vi "Manual Assembly DB.vi"() -> ()   [LabVIEW 2021]
uses:
  Classes/Routine/Routine Enum.ctl
  Classes/Assembly/Database Entry/Database Entry.lvclass
  Classes/Assembly/Assembly Run.lvclass
  Classes/Workspace/Fixture Enum.ctl
  <vilib>/Utility/file.llb/Read Delimited Spreadsheet (string).vi
  SubVIs/PUT_region.vi
  SubVIs/component_tray_region.vi
  SubVIs/assembly_tray_region.vi
  Classes/Workspace/Fixture.lvclass
  Classes/Controller/Controller.lvclass
  <vilib>/JDP Science/JDP Science Common Utilities/JDP Utility.lvlib
  Classes/Routine/Routine.lvclass
panel:
  out "Assembly Type":string[](array[string])
  out "Assembly tray region":dbl
  out "Component tray region":dbl
  out "PUT Region":dbl
  in  "Clear All":bool
  in  "Assemble":bool
  in  "Pick and Place":bool
  in  "Dispense glue":bool
  in  "Go":bool
  in  "Routine":T1=enum."Dispense Epoxy"
  in  "Update":bool
  in  "Stage":i32(listbox)=-1
  in  "Stop":bool
  in  "Remove":bool
  in  "Add":bool
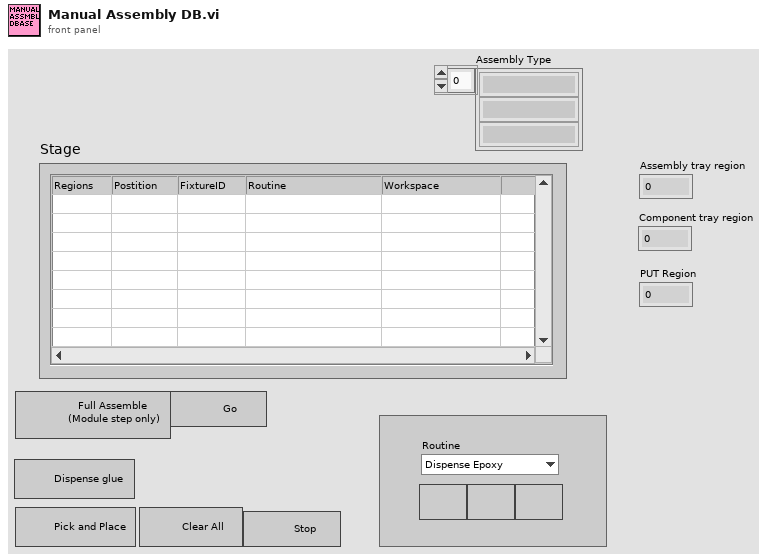
[diagram p1: front panel]
types:
  T1 = typedef "Routine.lvclass/Routine Enum.ctl" = enum16{"Primary Pick Up", "Secondary Pick Up", "Put Down All", "Secure Syringe", "Release Syringe", "Dispense Epoxy", "Pick Up All", "Put Down Secondary", "Full Assembly"}
  T2 = typedef "Fixture.lvclass/Fixture Enum.ctl" = enum16{"Assembly Tray", "Syringe Space", "Component", "Pick Up Tool", "Current Position"}
  T3 = typedef "File Paths.ctl" = cluster{"Glue Pattern Folder":path, "Carrier Tray Folder":path, "Pick Up Tool Fixture Folder":path, "Components Folder":path, "Bellows Tool Offset.txt":path, "Pick Up Tool Offset.txt":path, "Dispense Tip Offset.txt":path, "Log Files":path, "Gantry Assembly Map.txt":path, "Syringe and offset map.txt":path, "Controllers Folder":path, "Local dbase config":path}
  T4 = cluster{"Fixture ID":dbl, "Position":dbl, "Thickness":dbl}[]
  T5 = typedef "Controller.lvclass/Controllers.ctl" = cluster{"I-O.lvclass":refnum<class "I-O.lvclass">, "Gantry":refnum<k24>, "Dispenser":refnum<visa-resource-name>}
  T6 = cluster{"Fixture ID":dbl, "Position":dbl, "Thickness":dbl}
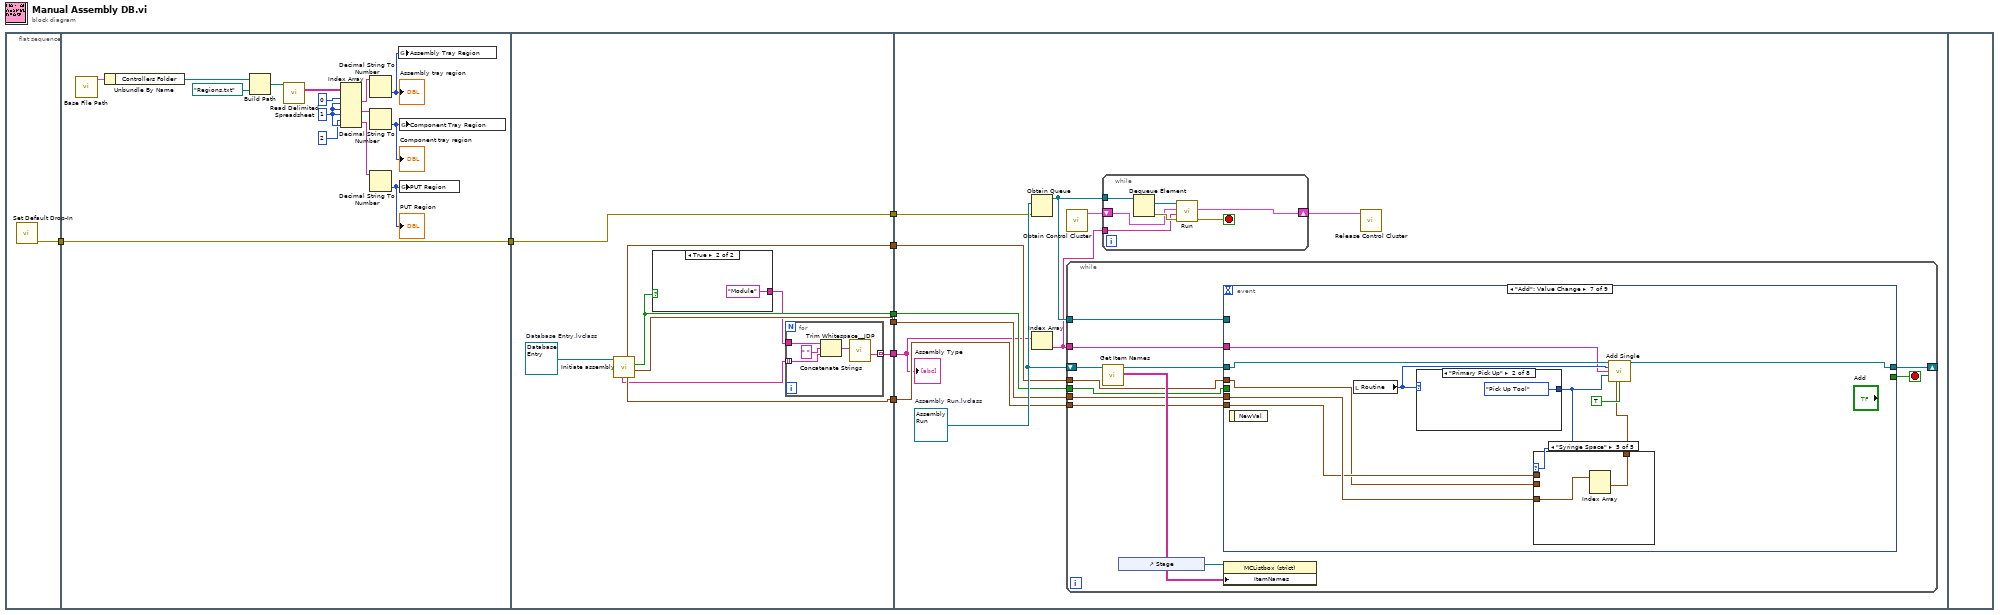
[diagram p0: block diagram]
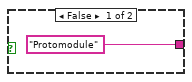
[diagram p2: hidden frame]
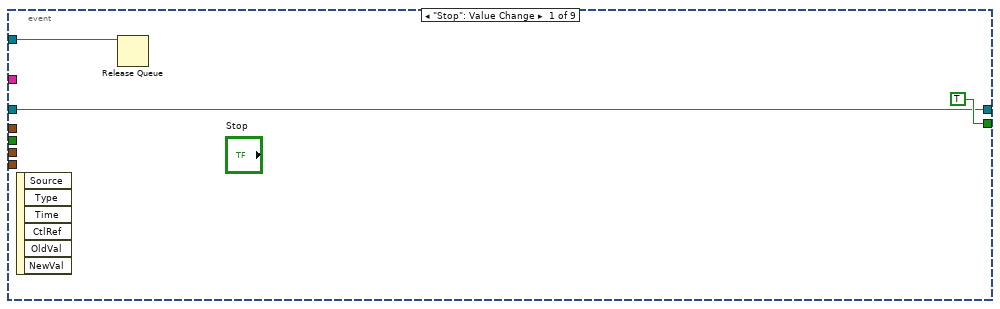
[diagram p3: hidden frame]
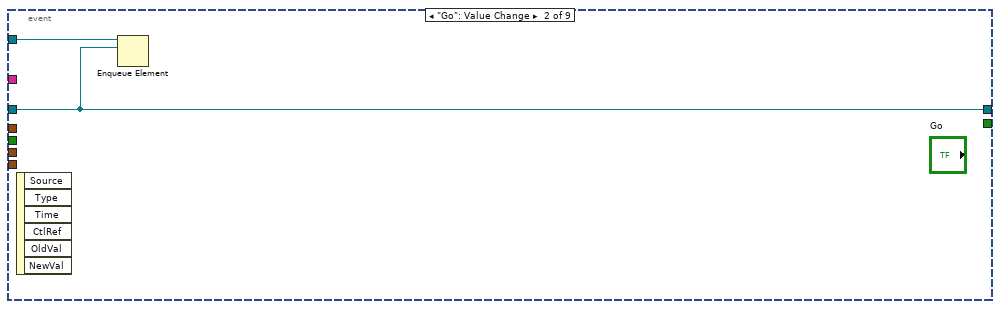
[diagram p4: hidden frame]
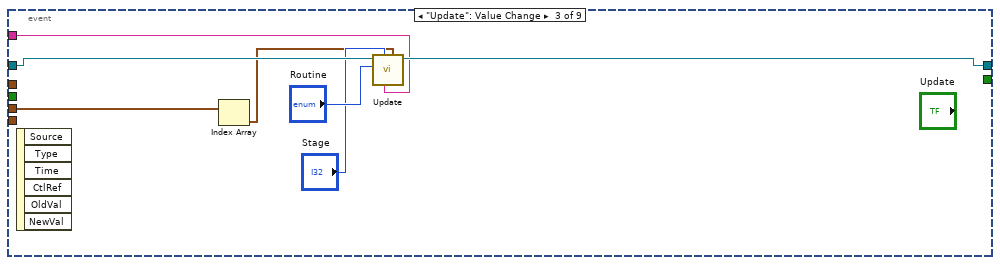
[diagram p5: hidden frame]
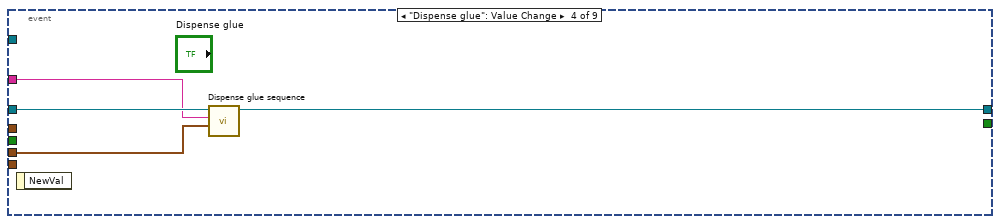
[diagram p6: hidden frame]
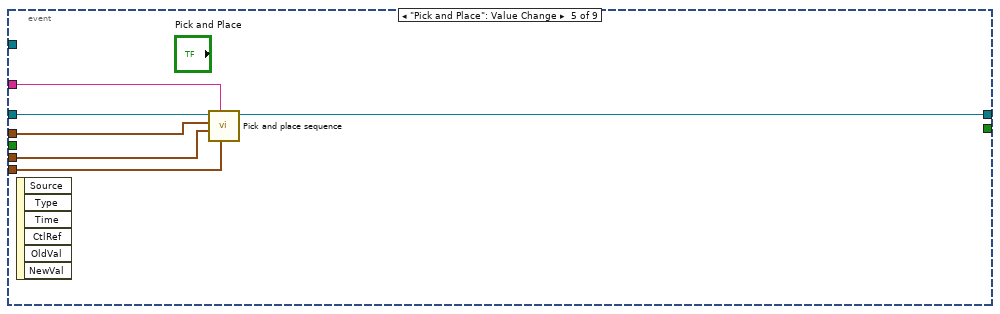
[diagram p7: hidden frame]
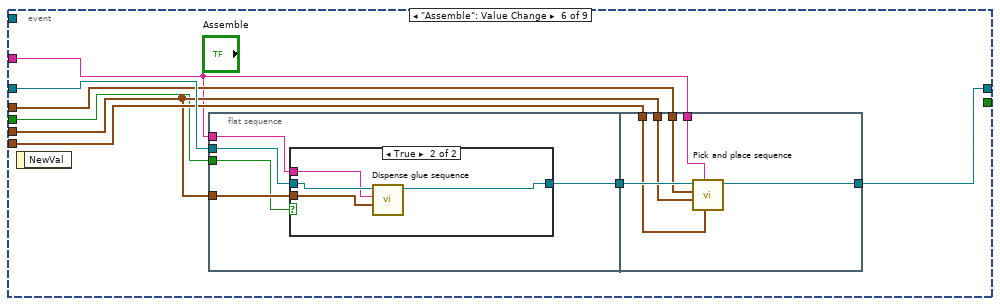
[diagram p8: hidden frame]
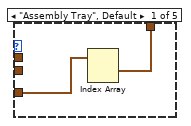
[diagram p10: hidden frame]
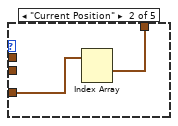
[diagram p11: hidden frame]
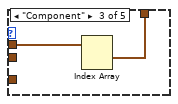
[diagram p12: hidden frame]
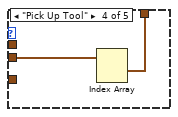
[diagram p13: hidden frame]
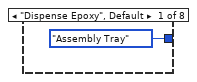
[diagram p14: hidden frame]
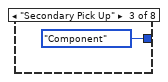
[diagram p15: hidden frame]
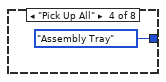
[diagram p16: hidden frame]
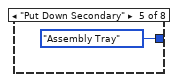
[diagram p17: hidden frame]
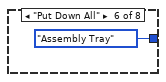
[diagram p18: hidden frame]
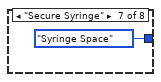
[diagram p19: hidden frame]
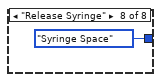
[diagram p20: hidden frame]
diagram:
  n1 = flat-sequence {
    tunnel: [w9] -> w6
    tunnel: [w10] -> w7
    tunnel: w6 -> [w10]
    tunnel: [w32] -> w8
    tunnel: w7 -> [w32]
    tunnel: [w31] -> w5
    tunnel: [w30] -> w4
    tunnel: [w29] -> w3
    tunnel: [w28] -> w2
    tunnel: [w25] -> w1
    tunnel: w8 -> [w47]
    tunnel: w5 -> [w46]
    tunnel: w4 -> [w45]
    tunnel: w3 -> [w44]
    tunnel: w2 -> [w43]
    tunnel: w1 -> [w42]
    frame #0 {
      n2 = call "Set Default Drop-In.vi"() -> ("error out"=w9:errorcluster)  [unwired: 11 in]
    }
    frame #1 {
      w13 = 1 ("disabled index (col)")
      n3 = call "Base File Path.vi"() -> ("Paths Out"=w24:T3)  [unwired: 11 in]
      n4 = Unbundle By Name(w24) -> ("Controllers Folder"=w22:path)
      n5 = Build Path(base path=w22, name or relative path=path "Regions.txt") -> (appended path=w23:path)
      n6 = call-poly <vilib>:"Read Delimited Spreadsheet.vi"("file path (dialog if empty)"=w23) -> ("all rows"=w11:string[][])  [unwired: 9 in, 5 out]
      n7 = Index Array(array=w11, index (row) #1=0 ("index (row)"), index (col) #1=w13, index (row) #2=w13, index (col) #2=w13, index (row) #3=2 ("disabled index (row)"), index (col) #3=w13) -> (element #1=w16:string, element #2=w15:string, element #3=w17:string)
      n8 = Decimal String To Number(string=w16) -> (number=w19:i32)  [unwired: 2 in, 1 out]
      "Assembly tray region" <- w19
      n9 = Decimal String To Number(string=w15) -> (number=w20:i32)  [unwired: 2 in, 1 out]
      "Component tray region" <- w20
      n10 = Decimal String To Number(string=w17) -> (number=w18:i32)  [unwired: 2 in, 1 out]
      "PUT Region" <- w18
      n11 = global write "assembly_tray_region.vi" "Assembly Tray Region"(w19) -> ()
      n12 = global write "component_tray_region.vi" "Component Tray Region"(w20) -> ()
      n13 = global write "PUT_region.vi" "PUT Region"(w18) -> ()
    }
    frame #2 {
      w33 = refnum<class "Database Entry.lvclass"> refnum  # Database Entry.lvclass
      n14 = call "Initiate assembly.vi"("Database Entry in"=w33) -> ("Assembly Settings"=w29:T4, "Module?"=w28:bool, "Component Settings"=w31:T4, "PUT Settings"=w30:T4, "Assembly Type"=w27:string[])  [unwired: 4 in, 2 out]
      n15 = case shown="True" w28 {
        tunnel: ["Protomodule" "Module"] -> w26
        frame False {
        }
        frame True {
        }
      }
      n16 = for {
        tunnel: w27 -> [w36] mode=indexing
        tunnel: w26 -> [w38]
        tunnel: [w34] -> w25 mode=indexing
        n17 = Concatenate Strings(w38, " " ("string"), w36) -> (w35:string)
        n18 = call <vilib>:"Trim Whitespace__JDP.vi"("String in"=w35) -> ("String out"=w34:string)  [unwired: 6 in]
      }
    }
    frame #3 {
      w49 = refnum<class "Assembly Run.lvclass"> refnum  # Assembly Run.lvclass
      n19 = Obtain Queue(element data type=w49, error in (no error)=w47) -> (queue out=w51:refnum<queue>)  [unwired: 3 in, 2 out]
      n20 = Index Array(array=w42) -> (element=w41:string)  [unwired: 1 in]
      n21 = call "Obtain Control Cluster.vi"() -> ("Control Out"=w48:T5)  [unwired: 11 in]
      n22 = while {
        shift-right: [w57] -> _
        shift-left: w49 -> [w59]
        tunnel: w51 -> [w62]
        tunnel: w46 -> [w56]
        tunnel: w45 -> [w55]
        tunnel: w44 -> [w54]
        tunnel: w43 -> [w53]
        tunnel: w41 -> [w52]
        stop <- w63 stop-if-true
        n23 = call "Get Item Names.vi"("Assembly Run in"=w59) -> ("Item names"=w61:string[][], "Assembly Run out"=w58:refnum<class "Assembly Run.lvclass">)  [unwired: 8 in, 1 out]
        n24 = control-ref of="Stage"() -> (w60:refnum<vi>)
        n25 = event shown="[6] \"Add\": Value Change" {
          selector: _ -> [_ _ _ _ _ _ _ _ _]
          dyn-events: _ -> [_ _ _ _ _ _ _ _ _]
          timeout: _ -> [_ _ _ _ _ _ _ _ _]
          tunnel: [TRUE _ _ _ _ _ _ _ _] -> w63
          tunnel: w58 -> [w65 w67 w75 w79 w85 w93 w118 w140 _]
          tunnel: [w65 w67 w74 w78 w84 w92 w119 w139 w144] -> w57
          tunnel: w62 -> [w64 w68 _ _ _ _ _ _ w143]
          tunnel: w56 -> [_ _ _ _ w81 w89 w111 _ _]
          tunnel: w55 -> [_ _ _ _ w83 w90 w110 _ _]
          tunnel: w54 -> [_ _ w70 w77 w80 w88 w114 _ _]
          tunnel: w53 -> [_ _ _ _ _ w87 _ _ _]
          tunnel: w52 -> [_ _ w71 w76 w82 w86 w116 _ _]
          event "Stop": Value Change {
            n26 = event-data() -> ()  [unwired: 1 in, 6 out]
            n27 = Release Queue(queue=w64) -> ()  [unwired: 2 in, 3 out]
          }
          event "Go": Value Change {
            n28 = event-data() -> ()  [unwired: 1 in, 6 out]
            n29 = Enqueue Element(queue=w68, element=w67) -> ()  [unwired: 2 in, 3 out]
          }
          event "Update": Value Change {
            n30 = event-data() -> ()  [unwired: 1 in, 6 out]
            n31 = Index Array(array=w70) -> (element=w69:T6)  [unwired: 1 in]
            n32 = call "Update.vi"("Input Settings"=w69, "Assembly Type"=w71, "Row"="Stage", "Routine"="Routine", "Assembly Run in"=w75) -> ("Assembly Run out"=w74:refnum<class "Assembly Run.lvclass">)  [unwired: 5 in, 1 out]
          }
          event "Dispense glue": Value Change {
            n33 = event-data() -> ()  [unwired: 1 in, 1 out]
            n34 = call "Dispense glue sequence.vi"("Assembly Tray Settings Array"=w77, "Assembly Type"=w76, "Assembly Run in"=w79) -> ("Assembly Run out"=w78:refnum<class "Assembly Run.lvclass">)  [unwired: 7 in, 1 out]
          }
          event "Pick and Place": Value Change {
            n35 = event-data() -> ()  [unwired: 1 in, 6 out]
            n36 = call "Pick and place sequence.vi"("Component Tray map"=w81, "Assembly Type"=w82, "Assembly Tray map"=w80, "PUT map"=w83, "Assembly Run in"=w85) -> ("Assembly Run out"=w84:refnum<class "Assembly Run.lvclass">)  [unwired: 5 in, 1 out]
          }
          event "Assemble": Value Change {
            n37 = event-data() -> ()  [unwired: 1 in, 1 out]
            n38 = flat-sequence {
              tunnel: [w97] -> w91
              tunnel: w93 -> [w98]
              tunnel: w88 -> [w96]
              tunnel: w87 -> [w95]
              tunnel: w86 -> [w94]
              tunnel: [w108] -> w92
              tunnel: w91 -> [w109]
              tunnel: w88 -> [w107]
              tunnel: w90 -> [w106]
              tunnel: w89 -> [w105]
              tunnel: w86 -> [w104]
              frame #0 {
                n39 = case shown="True" w95 {
                  tunnel: w98 -> [w99 w103]
                  tunnel: [w99 w102] -> w97
                  tunnel: w96 -> [_ w101]
                  tunnel: w94 -> [_ w100]
                  frame False {
                  }
                  frame True {
                    n40 = call "Dispense glue sequence.vi"("Assembly Tray Settings Array"=w101, "Assembly Type"=w100, "Assembly Run in"=w103) -> ("Assembly Run out"=w102:refnum<class "Assembly Run.lvclass">)  [unwired: 7 in, 1 out]
                  }
                }
              }
              frame #1 {
                n41 = call "Pick and place sequence.vi"("Component Tray map"=w105, "Assembly Type"=w104, "Assembly Tray map"=w107, "PUT map"=w106, "Assembly Run in"=w109) -> ("Assembly Run out"=w108:refnum<class "Assembly Run.lvclass">)  [unwired: 5 in, 1 out]
              }
            }
          }
          event "Add": Value Change {
            n42 = event-data() -> ()  [unwired: 1 in, 1 out]
            n43 = local read "Routine"() -> (w117:T1)
            n44 = case shown="\"Primary Pick Up\"" w117 {
              tunnel: [Fixture_Enum."Assembly Tray" ("Fixture") Fixture_Enum."Pick Up Tool" ("Fixture") Fixture_Enum."Component" ("Fixture") Fixture_Enum."Assembly Tray" ("Fixture") Fixture_Enum."Assembly Tray" ("Fixture") Fixture_Enum."Assembly Tray" ("Fixture") Fixture_Enum."Syringe Space" ("Fixture") Fixture_Enum."Syringe Space" ("Fixture")] -> w112
              frame "Dispense Epoxy", Default {
              }
              frame "Primary Pick Up" {
              }
              frame "Secondary Pick Up" {
              }
              frame "Pick Up All" {
              }
              frame "Put Down Secondary" {
              }
              frame "Put Down All" {
              }
              frame "Secure Syringe" {
              }
              frame "Release Syringe" {
              }
            }
            n45 = case shown="\"Syringe Space\"" w112 {
              tunnel: w114 -> [w121 w123 _ _ w129]
              tunnel: [w120 w122 w125 w127 w128] -> w113
              tunnel: w111 -> [_ _ w124 _ _]
              tunnel: w110 -> [_ _ _ w126 _]
              frame "Assembly Tray", Default {
                n46 = Index Array(array=w121) -> (element #1=w120:T6)  [unwired: 2 in, 1 out]
              }
              frame "Current Position" {
                n47 = Index Array(array=w123) -> (element #1=w122:T6)  [unwired: 2 in, 1 out]
              }
              frame "Component" {
                n48 = Index Array(array=w124) -> (element #1=w125:T6)  [unwired: 2 in, 1 out]
              }
              frame "Pick Up Tool" {
                n49 = Index Array(array=w126) -> (element #1=w127:T6)  [unwired: 2 in, 1 out]
              }
              frame "Syringe Space" {
                n50 = Index Array(array=w129) -> (element #1=w128:T6)  [unwired: 2 in, 1 out]
              }
            }
            n51 = call-dynamic "Add Single.vi"("UI in"=w118, "Routine"=w117, "Assembly Type"=w116, "Fixture"=w112, "Input Settings"=w113, "Auto"=TRUE) -> ("UI out"=w119:refnum<class "Assembly Run.lvclass">)  [unwired: 8 in, 1 out]
          }
          event "Remove": Value Change {
            n52 = event-data() -> ()  [unwired: 1 in, 6 out]
            n53 = local read "Stage"() -> (w138:i32)
            n54 = call "Delete.vi"("Index"=w138, "Assembly In"=w140) -> ("Assembly Out"=w139:refnum<class "Assembly Run.lvclass">)  [unwired: 8 in, 1 out]
          }
          event "Clear All": Value Change {
            w144 = refnum<class "Assembly Run.lvclass"> refnum  # Assembly Run.lvclass
            n55 = event-data() -> ()  [unwired: 1 in, 6 out]
            n56 = Flush Queue(queue=w143) -> ()  [unwired: 1 in, 3 out]
            n57 = invoke on="Stage" class="MCListbox (strict)" method="Reinit To Default"() -> ()  [unwired: 3 in, 3 out]
            n58 = Build Array(FALSE) -> (w142:bool[])
            n59 = Array To Cluster(array=w142) -> ()  [unwired: 1 out]
          }
        }
        n60 = property class="MCListbox (strict)"(reference=w60, "ItemNames"=w61) -> ()  [unwired: 1 in, 2 out]
      }
      n61 = while {
        tunnel: w51 -> [w151]
        shift-right: [w146] -> w50
        shift-left: w48 -> [w147]
        tunnel: w41 -> [w145]
        stop <- w148 stop-if-true
        n62 = Dequeue Element(queue=w151) -> (element=w150:refnum<class "Assembly Run.lvclass">, error out=w149:errorcluster)  [unwired: 2 in, 2 out]
        n63 = call-dynamic "Run.vi"("error in (no error)"=w149, "Assembly Type"=w145, "Control In"=w147, "Assembly In"=w150) -> ("error out"=w148:errorcluster, "Control Out"=w146:T5)  [unwired: 5 in, 1 out]
      }
      n64 = call "Release Control Cluster.vi"("output cluster"=w50) -> ()  [unwired: 11 in]
      "Assembly Type" <- w42
    }
    frame #4 {
    }
  }
